vi "lab4_sim_cp_ofdm_transceiver.vi"() -> ()   [LabVIEW 2014]
uses:
  <vilib>/vision/Image Controls.llb/IMAQ Image.ctl
  <vilib>/Analysis/2dsp.llb/Inverse Complex FFT.vi
  <vilib>/Analysis/2dsp.llb/Complex FFT.vi
  <vilib>/Analysis/5stat.llb/RMS (DBL).vi
  <vilib>/addons/Modulation/Digital/General/MT Generate QAM System Parameters(M).vi
  <vilib>/addons/Modulation/Digital/General/MT Map Bits to QAM Symbols.vi
  <vilib>/gmath/statdist.llb/Normal Random.vi
  <vilib>/addons/Modulation/Digital/General/MT Map QAM Symbols to Bits.vi
  <vilib>/Analysis/NI_AALPro.lvlib
  <vilib>/addons/Modulation/niDMT.lvlib
  <vilib>/gmath/NI_Gmath.lvlib
panel:
  out "length 2":i32
  out "length":i32
  out "frame":T1(plugin-control)
  out "string":string
  out "number":u32
  out "pilot channel gain":dbl[](graph)
  out "pilot channel gain":dbl[](graph)
  out "PAPR":dbl
  out "Error bits":i32
  out "Bit compare":bool[](array[boolean])
  out "BER":dbl
  in  "millisecond multiple":u32=20
  out "output bit stream 2":i8[](array[numeric]) caption="Transmit output bit stream"
  out "output bit stream":i8[](array[numeric]) caption="Received output bit stream"
  in  "M-QAM (16)":i32=16
  out "Transmit FFT (Magnitude)":dbl[](graph)
  out "Receiver FFT (Magnitude)":dbl[](graph)
  out "RX constellation":cdb[](graph)
  in  "pilot carrier":i32=32
  in  "message carrier":i32=120
  out "eb/n0 (dB)":dbl=38.96307662438871
  in  "Symbol energy es/n0(db)":dbl=50.0 format="%#_13g"
  in  "stop":bool
  in  "cyclic prefix":i32=64
  in  "FFT size":i32=256
  in  "ofdm symbols":i32=10
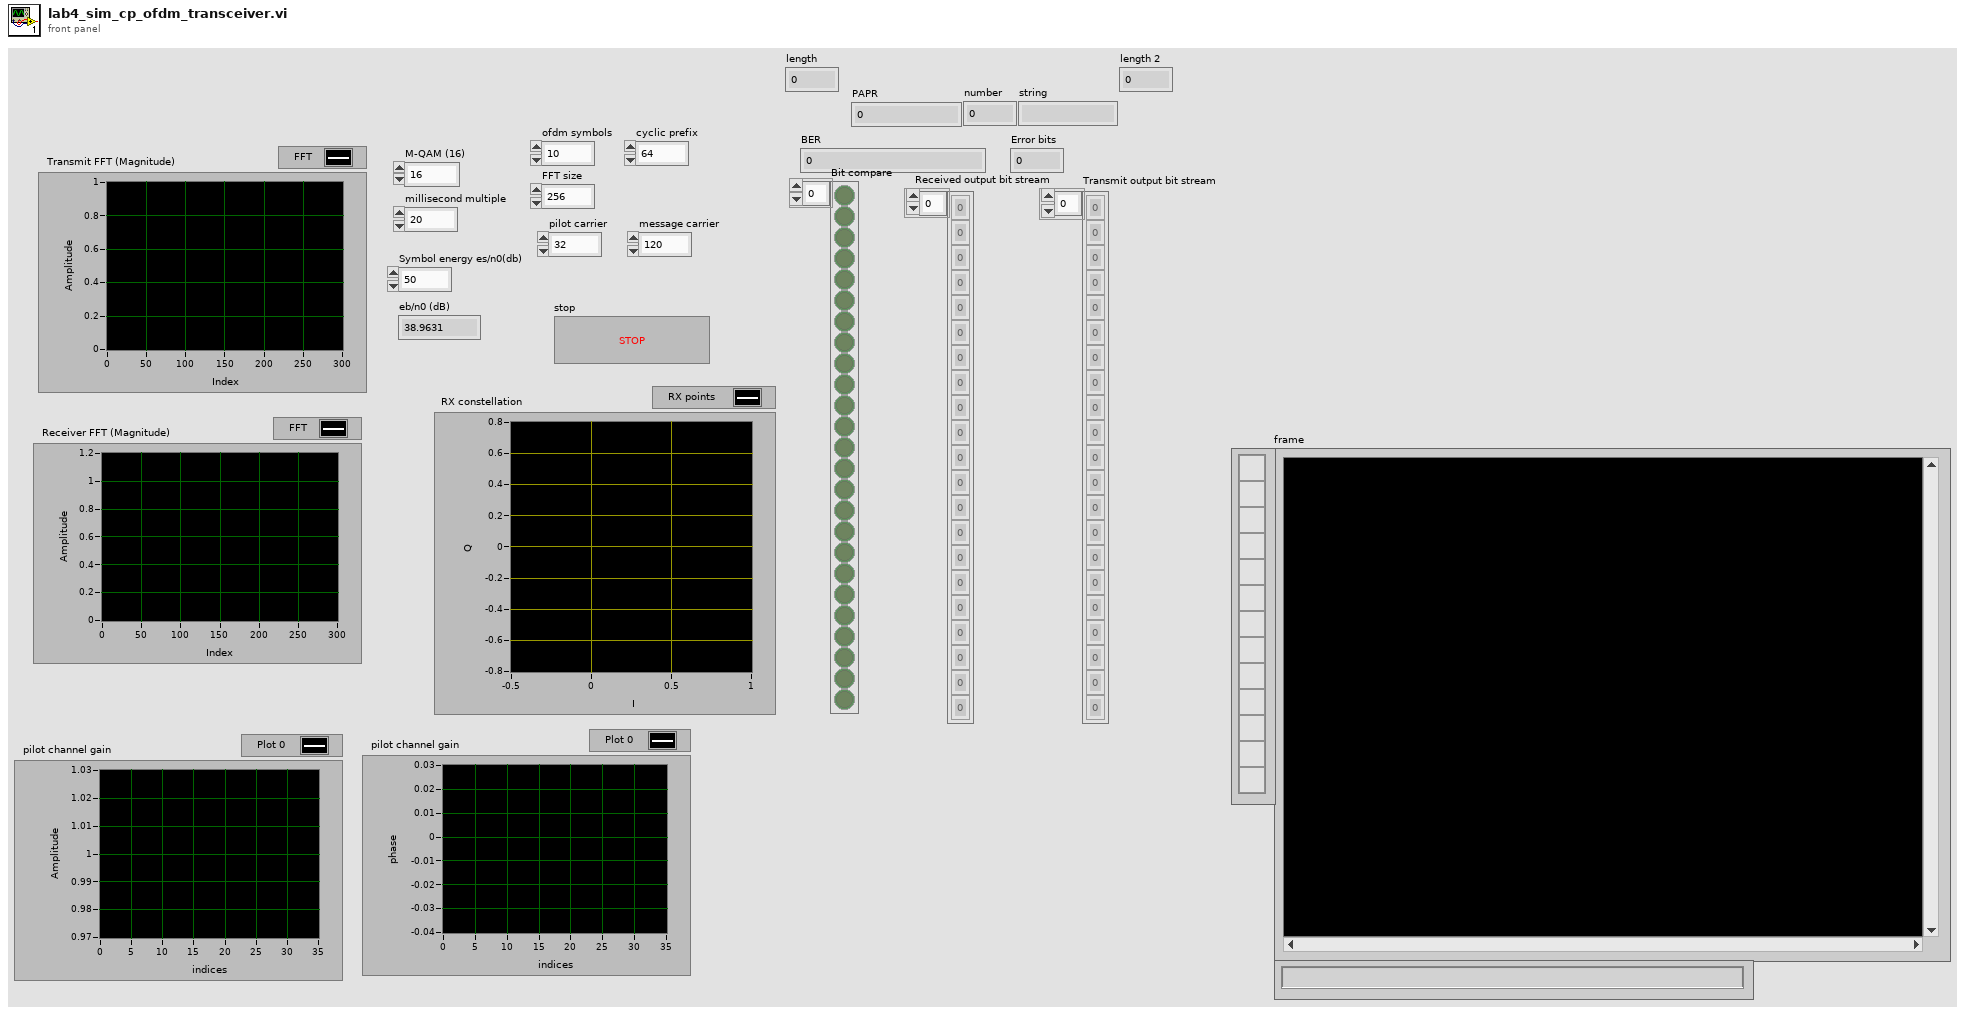
[diagram p1: front panel]
types:
  T1 = typedef "IMAQ Image.ctl" = refnum<image>
  T2 = cluster{"samples per symbol (16)":i32, "symbol map":cdb[]}
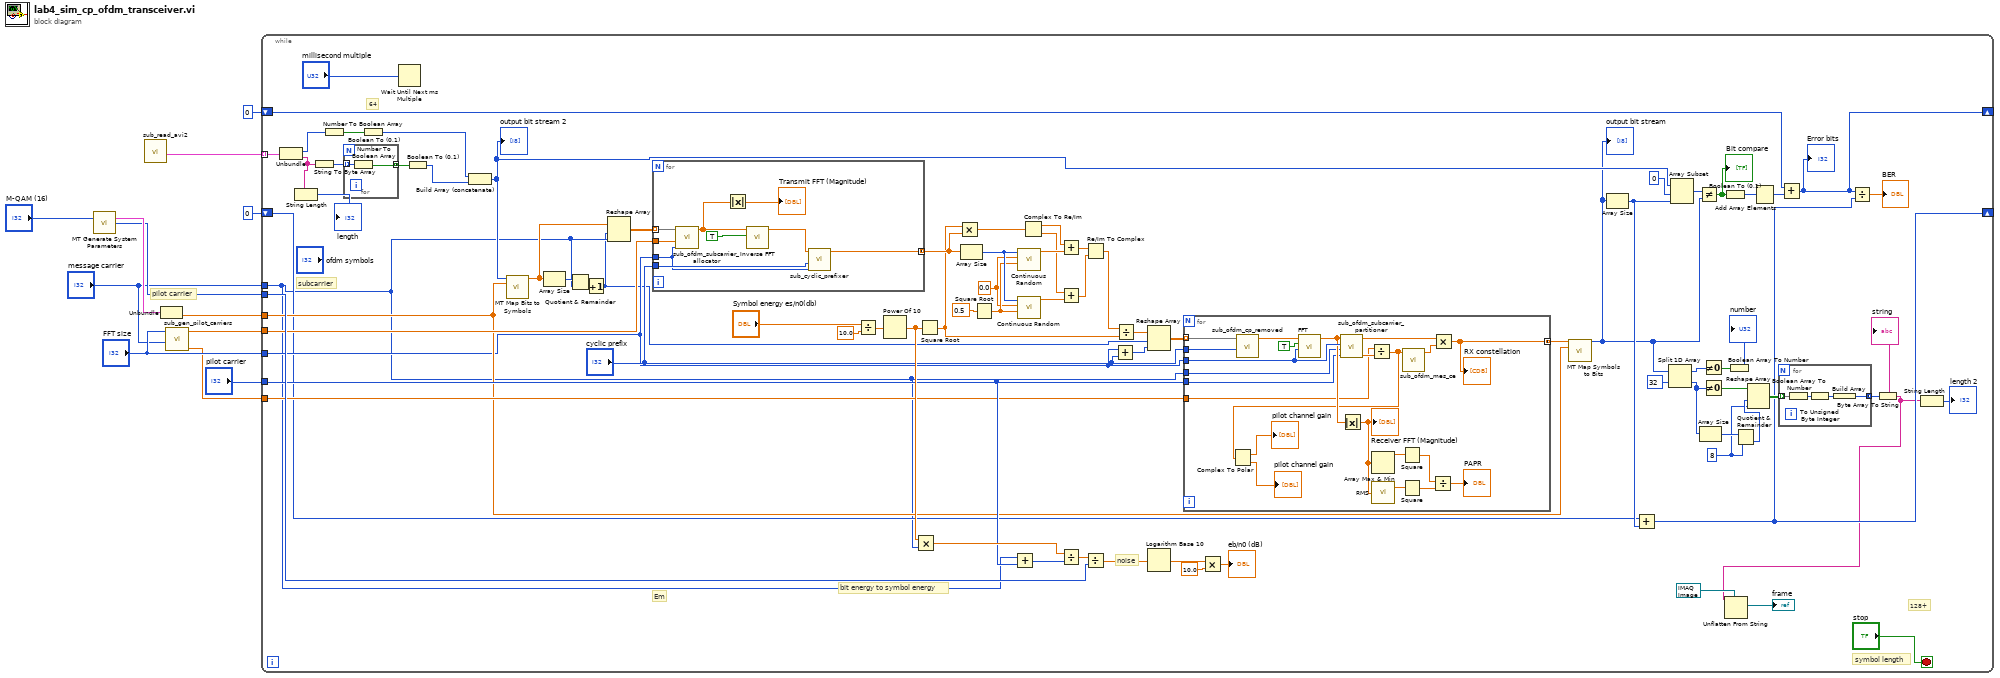
[diagram p0: block diagram]
diagram:
  # "pilot carrier"
  n1 = call-poly <vilib>:"MT Generate System Parameters.vi"("M-QAM (16)"="M-QAM (16)") -> ("QAM system parameters"=w10:T2, "bits per symbol"=w8:i32)  [unwired: 12 in, 1 out]
  n2 = call "sub_read_avi2.vi"() -> ("frames"=w1:cluster{i32, "Data String":string}[])  [unwired: 10 in, 1 out]
  n3 = Unbundle(w10) -> ("symbol map"=w9:cdb[])  [unwired: 1 out]
  n4 = call "sub_gen_pilot_carriers.vi"("message carrier"="message carrier", "FFT size"="FFT size") -> ("RX pilot carriers"=w3:cdb[], "TX pilot carriers"=w2:cdb[])  [unwired: 8 in]
  n5 = while {
    tunnel: w8 -> [w81]
    tunnel: w2 -> [w77]
    tunnel: "pilot carrier" -> [w75]
    tunnel: "message carrier" -> [w20]
    tunnel: "FFT size" -> [w65]
    tunnel: w3 -> [w74]
    tunnel: w9 -> [w73]
    shift-right: [w47] -> _
    shift-left: 0 -> [w50]
    shift-right: [w24] -> _
    shift-left: 0 -> [w48]
    tunnel: w1 -> [w43] mode=indexing
    stop <- "stop" stop-if-true
    w26 = 8 ("y")
    w44 = 0.0 ("mean")
    # "128+"
    # "symbol length"
    # "bit energy to symbol energy"
    # "noise"
    # "subcarrier"
    # "Em"
    # "64"
    n6 = Unbundle(w43) -> (w40:i32, "Data String"=w17:string)
    n7 = String Length(string=w17) -> (length=→"length":i32)
    n8 = String To Byte Array(string=w17) -> (unsigned byte array=w42:u8[])
    n9 = Number To Boolean Array(number=w40) -> (Boolean array=w39:bool[])
    n10 = for {
      tunnel: w42 -> [w99] mode=indexing
      tunnel: [w98] -> w41 mode=concatenating
      n11 = Number To Boolean Array(number=w99) -> (Boolean array=w98:bool[])
    }
    n12 = Boolean To (0,1)(Boolean=w39) -> (0, 1=w37:i16[])
    n13 = Wait Until Next ms Multiple(millisecond multiple="millisecond multiple") -> ()  [unwired: 1 out]
    n14 = Boolean To (0,1)(Boolean=w41) -> (0, 1=w38:i16[])
    n15 = Build Array (concatenate)(w37, w38) -> (w36:i16[])
    "output bit stream 2" <- w36
    n16 = call-poly <vilib>:"MT Map Bits to Symbols.vi"("input bit stream"=w36, "symbol map"=w73) -> ("symbols"=w79:cdb[])  [unwired: 12 in, 1 out]
    n17 = Array Size(array=w79) -> (size(s)=w93:i32)
    n18 = Quotient & Remainder(x=w93, y=w20) -> (floor(x/y)=w21:i32)  [unwired: 1 out]
    n19 = Increment(x=w21) -> (x+1=w13:i32)
    n20 = Reshape Array(w79, w13, w20) -> (w78:cdb[][])
    n21 = for {
      tunnel: w78 -> [w130] mode=indexing
      tunnel: w77 -> [w129]
      tunnel: w65 -> [w125]
      tunnel: "cyclic prefix" -> [w126]
      tunnel: [w124] -> w62 mode=concatenating
      n22 = call "sub_ofdm_subcarrier_allocator.vi"("fft size"=w125, "pilot symbol"=w129, "message symbol"=w130) -> ("OFDM symbol"=w123:cdb[])  [unwired: 8 in]
      n23 = Absolute Value(x=w123) -> (abs(x)=→"Transmit FFT (Magnitude)":dbl[])
      n24 = call-poly <vilib>:"Inverse FFT.vi"("shift?"=TRUE, "FFT {X}"=w123) -> ("X"=w127:cdb[])  [unwired: 8 in, 1 out]
      n25 = call "sub_cyclic_prefixer.vi"("FFT size"=w125, "CP length"=w126, "time_samples"=w127) -> ("cp ofdm symbol"=w124:cdb[])  [unwired: 8 in]
    }
    n26 = Divide(x="Symbol energy es/n0(db)", y=10.0) -> (x/y=w88:dbl)
    n27 = Power Of 10(x=w88) -> (10^x=w84:dbl)
    n28 = Multiply(x=w84, y=w20) -> (x*y=w83:dbl)
    n29 = Square Root(x=w84) -> (sqrt(x)=w53:dbl)
    n30 = Multiply(x=w53, y=w62) -> (x*y=w63:cdb[])
    n31 = Array Size(array=w62) -> (size(s)=w61:i32)
    n32 = Square Root(x=0.5 ("std")) -> (sqrt(x)=w45:dbl)
    n33 = Add(x=w20, y=w75) -> (x+y=w76:i32)
    n34 = call-poly <vilib>:"Continuous Random.vi"("std"=w45, "mean"=w44, "samples"=w61) -> ("normal random data"=w59:dbl[])  [unwired: 7 in, 1 out]
    n35 = call-poly <vilib>:"Continuous Random.vi"("std"=w45, "mean"=w44, "samples"=w61) -> ("normal random data"=w57:dbl[])  [unwired: 7 in, 1 out]
    n36 = Complex To Re/Im(x + iy=w63) -> (x=w60:dbl[], y=w58:dbl[])
    n37 = Add(x=w60, y=w59) -> (x+y=w56:dbl[])
    n38 = Add(x=w58, y=w57) -> (x+y=w55:dbl[])
    n39 = Divide(x=w83, y=w76) -> (x/y=w82:dbl)
    n40 = Re/Im To Complex(1:w55, 2:w56) -> (0:w54:cdb[])
    n41 = Divide(x=w82, y=w81) -> (x/y=w80:dbl)
    n42 = Add(x=w65, y="cyclic prefix") -> (x+y=w64:i32)
    n43 = Divide(x=w54, y=w53) -> (x/y=w52:cdb[])
    n44 = Reshape Array(w52, w13, w64) -> (w67:cdb[][])
    n45 = Logarithm Base 10(1:w80) -> (0:w87:dbl)
    n46 = for {
      tunnel: w67 -> [w121] mode=indexing
      tunnel: "cyclic prefix" -> [w120]
      tunnel: w65 -> [w117]
      tunnel: [w115] -> w68 mode=concatenating
      tunnel: w20 -> [w113]
      tunnel: w75 -> [w112]
      tunnel: w74 -> [w109]
      n47 = call "sub_ofdm_cp_removed.vi"("CP length"=w120, "time ofdm symbol"=w121) -> ("cp removed ofdm symbol"=w118:cdb[])  [unwired: 9 in]
      n48 = call-poly <vilib>:"FFT.vi"("FFT size"=w117, "shift?"=TRUE, "X"=w118) -> ("FFT {X}"=w114:cdb[])  [unwired: 7 in, 1 out]
      n49 = call "sub_ofdm_subcarrier_partitioner.vi"("pilot carrier"=w112, "message carrier"=w113, "FFT size"=w117, "received symbol"=w114) -> ("pilot subcarriers"=w116:cdb[], "message subcarriers"=w110:cdb[])  [unwired: 6 in]
      n50 = Absolute Value(x=w114) -> (abs(x)=w108:dbl[])
      "Receiver FFT (Magnitude)" <- w108
      n51 = Divide(x=w109, y=w116) -> (x/y=w102:cdb[])
      n52 = Complex To Polar(r * e^(i*theta)=w102) -> (r=→"pilot channel gain":dbl[], theta=→"pilot channel gain":dbl[])
      n53 = Array Max & Min(array=w108) -> (max value=w107:dbl)  [unwired: 3 out]
      n54 = call-poly <vilib>:"RMS.vi"("X"=w108) -> ("rms value"=w106:dbl)  [unwired: 1 out]
      n55 = Square(x=w107) -> (x^2=w105:dbl)
      n56 = Square(x=w106) -> (x^2=w104:dbl)
      n57 = call "sub_ofdm_mes_ce.vi"("ZF channel estimates"=w102) -> ("interpolated mes carrier CE"=w111:cdb[])  [unwired: 10 in]
      n58 = Divide(x=w105, y=w104) -> (x/y=→"PAPR":dbl)
      n59 = Multiply(x=w110, y=w111) -> (x*y=w115:cdb[])
      "RX constellation" <- w115
    }
    n60 = Multiply(x=w87, y=10.0) -> (x*y=→"eb/n0 (dB)":dbl)
    n61 = call-poly <vilib>:"MT Map Symbols to Bits.vi"("symbols"=w68, "symbol map"=w73) -> ("output bit stream"=w34:i8[])  [unwired: 12 in, 1 out]
    "output bit stream" <- w34
    n62 = Array Size(array=w34) -> (size(s)=w49:i32)
    n63 = Add(x=w48, y=w49) -> (x+y=w24:i32)
    n64 = Split 1D Array(array=w34, index=32) -> (first subarray=w32:i8[], second subarray=w29:i8[])
    n65 = Array Subset(array=w36, index=0, length=w49) -> (w35:i16[])
    n66 = Not Equal?(x=w35, y=w34) -> (x != y?=w72:bool[])
    "Bit compare" <- w72
    n67 = Array Size(array=w29) -> (size(s)=w28:i32)
    n68 = Not Equal To 0?(x=w32) -> (x != 0?=w31:bool[])
    n69 = Not Equal To 0?(x=w29) -> (x != 0?=w30:bool[])
    n70 = Boolean To (0,1)(Boolean=w72) -> (0, 1=w71:i16[])
    n71 = Boolean Array To Number(Boolean array=w31) -> (number=→"number":u32)
    n72 = Quotient & Remainder(x=w28, y=w26) -> (floor(x/y)=w27:i32)  [unwired: 1 out]
    n73 = Reshape Array(w30, w27, w26) -> (w25:bool[][])
    n74 = Add Array Elements(numeric array=w71) -> (sum=w51:i16)
    n75 = for {
      tunnel: w25 -> [w97] mode=indexing
      tunnel: [w95] -> w23 mode=concatenating
      n76 = Boolean Array To Number(Boolean array=w97) -> (number=w96:u32)
      n77 = To Unsigned Byte Integer(number=w96) -> (unsigned 8bit integer=w94:u8)
      n78 = Build Array(w94) -> (w95:u8[])
    }
    n79 = Add(x=w50, y=w51) -> (x+y=w47:i32)
    "Error bits" <- w47
    n80 = Divide(x=w47, y=w24) -> (x/y=→"BER":dbl)
    n81 = Byte Array To String(unsigned byte array=w23) -> (string=w15:string)
    "string" <- w15
    n82 = Unflatten From String(type=T1 refnum ("frame 2"), binary string=w15) -> (value=→"frame":T1)  [unwired: 3 in, 2 out]
    n83 = String Length(string=w15) -> (length=→"length 2":i32)
  }
